vi "DO Control.vi"(9 "DI List_280":string[](array[string]), 10 "s":bool, 11 "Control":string[](array[string])) -> (0 "Feedback":i32[](array[numeric]), 1 "Parameter (Out)":u8 caption="Poll Type", 2 "Control Channel":i32[](array[numeric]), 3 "Poll Time (Out)":u32 caption="Poll Time (ms)" max=600000 step=100, 4 "Tab Control 2":enum32{"Output", "Input"}(ring), 5 "Cancel":bool)   [LabVIEW 2015]
uses:
  Control Button/Exit.ctl
  Control Button/next.ctl
  Galobal variable_TI.vi
panel:
  out "Row":i32
  in  "s 2":bool
  out "Pokayoka Result":cluster{"Sensor Name":string, "Boolean":bool}[](array[cluster]) caption="Pokayoka Status"
  in  "Tab Control":enum32{"Output", "Input"}(tab)
  in  "Control Channel":i32[](listbox)=[7]
  in  "Control":bool
  in  "Feed Back Channel":i32[](listbox)=[0]
  in  "ok":T1
  in  "stop":T2
  # "Control Channel"
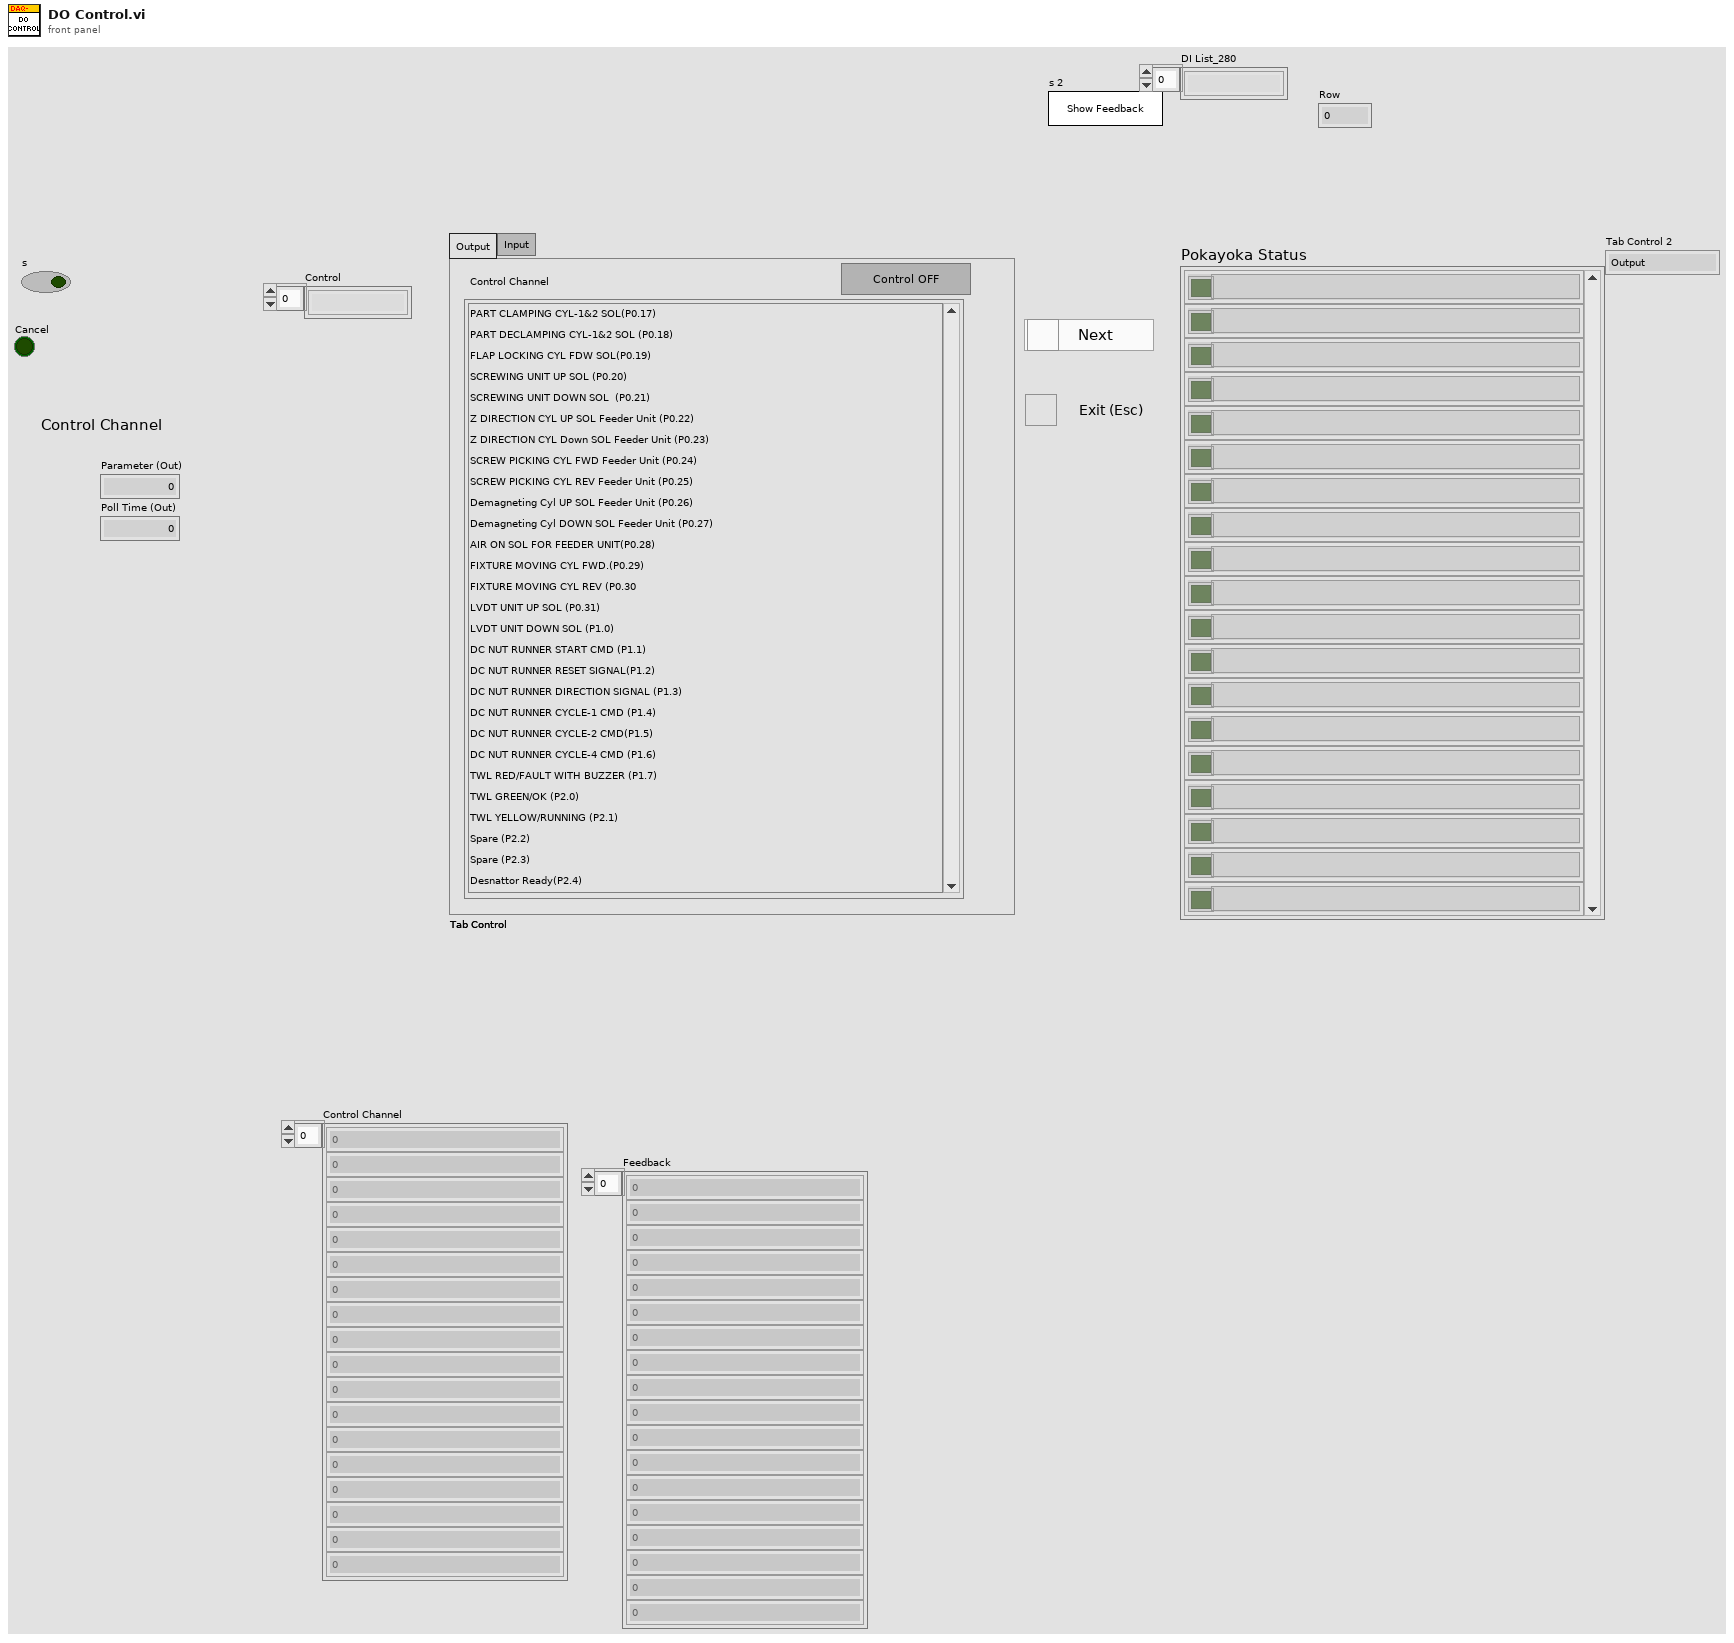
[diagram p1: front panel]
types:
  T1 = typedef "next.ctl" = bool
  T2 = typedef "Exit.ctl" = bool
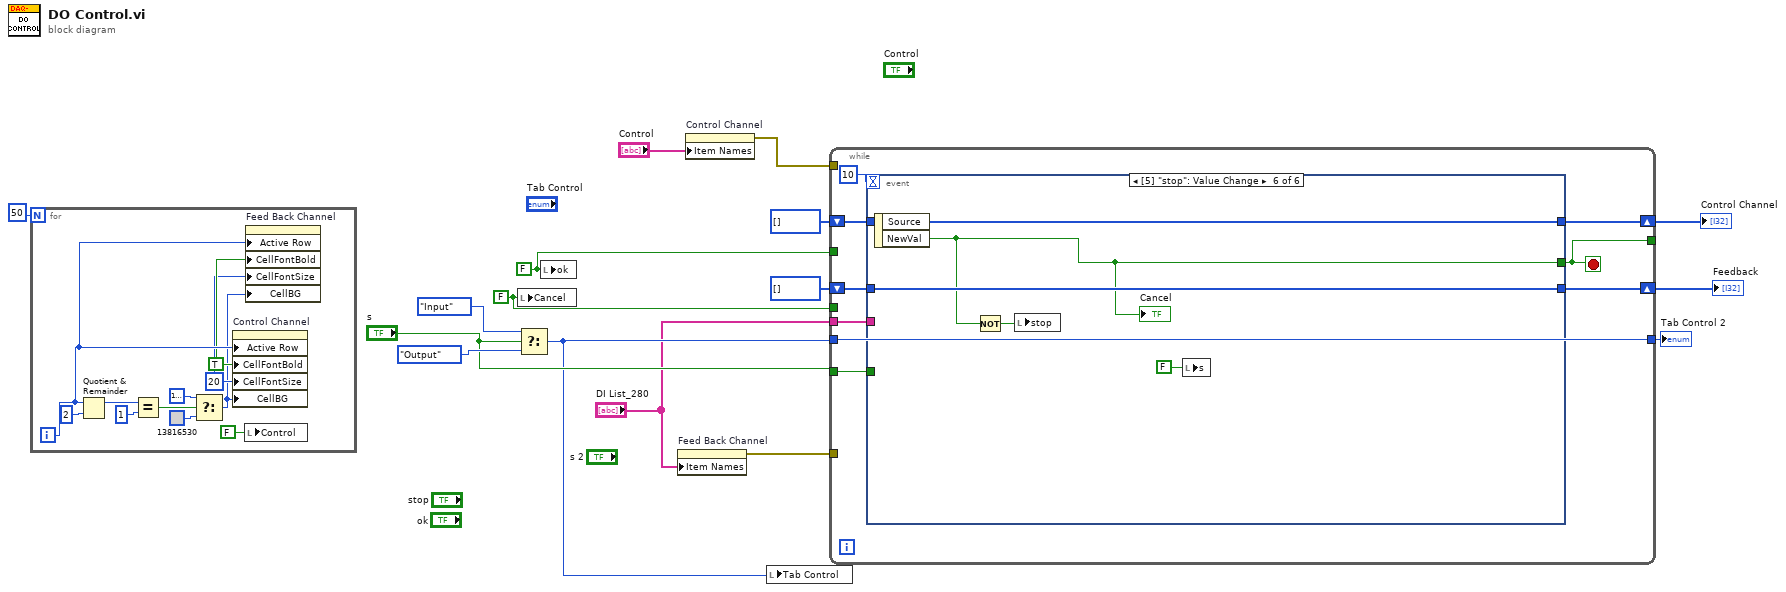
[diagram p0: block diagram]
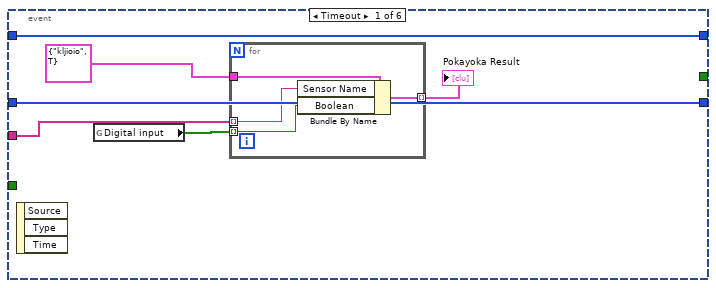
[diagram p2: hidden frame]
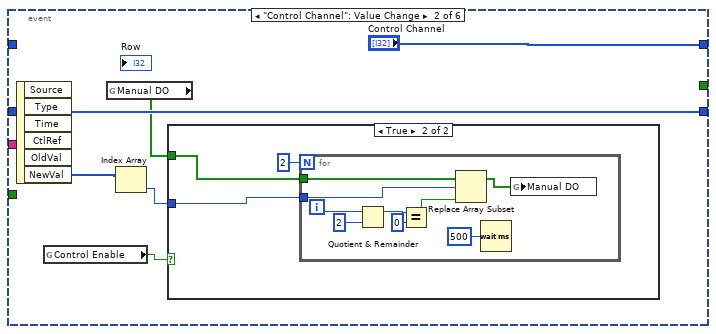
[diagram p3: hidden frame]
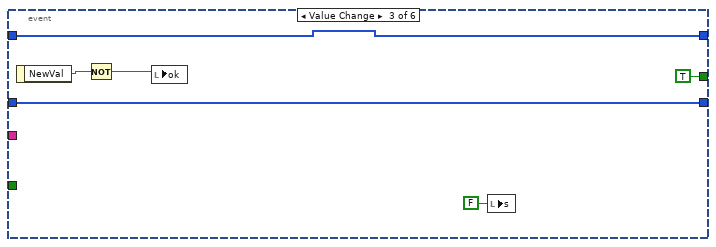
[diagram p5: hidden frame]
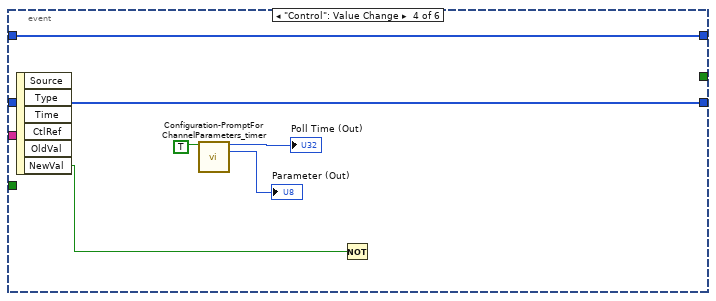
[diagram p6: hidden frame]
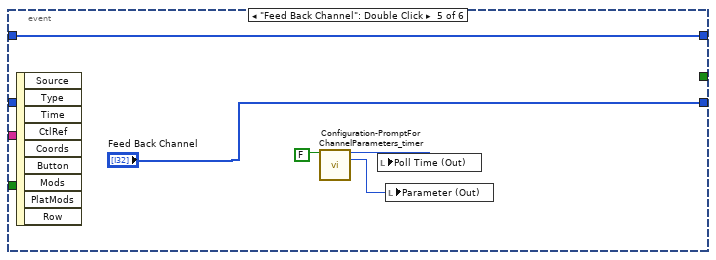
[diagram p7: hidden frame]
diagram:
  w9 = FALSE ("Cancel")
  w10 = FALSE ("ok")
  n1 = for {
    N: 50 -> [_]
    i -> [w21]
    w19 = u32 20 ("Active Row:Cell Font:Size")
    w20 = TRUE ("Active Row:Cell Font:Bold")
    n2 = Quotient & Remainder(x=w21, y=2) -> (x-y*floor(x/y)=w26:i32)  [unwired: 1 out]
    n3 = Equal?(x=w26, y=1) -> (x = y?=w24:bool)
    n4 = Select(t=u32 16777225 ("Color Box"), s=w24, f=u32 13816530 ("Color Box")) -> (s? t:f=w18:u32)
    n5 = property on="Control Channel" class="LstBox (strict)"("Active Row"=w21, "CellFontBold"=w20, "CellFontSize"=w19, "CellBG"=w18) -> ()  [unwired: 2 in, 2 out]
    n6 = local write "Control"(FALSE ("Control")) -> ()
    n7 = property on="Feed Back Channel" class="LstBox (strict)"("Active Row"=w21, "CellFontBold"=w20, "CellFontSize"=w19, "CellBG"=w18) -> ()  [unwired: 2 in, 2 out]
  }
  n8 = local write "Cancel"(w9) -> ()
  n9 = Select(t=enum32{"Output", "Input"}."Input" ("Tab Control"), s="s", f=enum32{"Output", "Input"}."Output" ("Tab Control")) -> (s? t:f=w12:enum32{"Output", "Input"})
  n10 = local write "ok"(w10) -> ()
  n11 = property on="Feed Back Channel" class="LstBox (strict)"("Item Names"="DI List_280") -> (error out=w7:errorcluster)  [unwired: 2 in, 1 out]
  n12 = property on="Control Channel" class="LstBox (strict)"("Item Names"="Control") -> (error out=w5:errorcluster)  [unwired: 2 in, 1 out]
  n13 = local write "Tab Control"(w12) -> ()
  n14 = while {
    tunnel: w12 -> [w28]
    tunnel: "s" -> [w35]
    tunnel: w10 -> [_]
    tunnel: [w33] -> _
    tunnel: w9 -> [_]
    shift-right: [w36] -> w16
    shift-left: i32[] [] ("Control Channel") -> [w32]
    shift-right: [w34] -> w11
    shift-left: i32[] [] ("Feed Back Channel") -> [w31]
    tunnel: "DI List_280" -> [w30]
    tunnel: w7 -> [_]
    tunnel: w5 -> [_]
    tunnel: [w28] -> w3
    stop <- w33 stop-if-true
    n15 = event shown="[5] \"stop\": Value Change" {
      selector: _ -> [_ _ _ _ _ _]
      dyn-events: _ -> [_ _ _ _ _ _]
      timeout: 10 -> [_ _ _ _ _ _]
      tunnel: [w42 "Control Channel" w69 w76 w78 w85] -> w36
      tunnel: [_ _ T2 TRUE ("NewVal") _ _ w83] -> w33
      tunnel: w35 -> [_ _ _ _ _ _]
      tunnel: [w41 w51 w68 w75 "Feed Back Channel" w84] -> w34
      tunnel: w32 -> [w42 _ w69 w76 w78 w85]
      tunnel: w31 -> [w41 w51 w68 w75 _ w84]
      tunnel: w30 -> [w38 _ _ _ _ _]
      event Timeout {
        n16 = event-data() -> ()  [unwired: 1 in, 3 out]
        n17 = global read "Galobal variable_TI.vi" "Digital input"() -> (w40:bool[])
        n18 = for {
          tunnel: w38 -> [w45] mode=indexing
          tunnel: cluster{"Sensor Name":string, "Boolean":bool} {"Sensor Name"="kljioio", "Boolean"=TRUE} ("Cluster") -> [w46]
          tunnel: [w44] -> w37 mode=indexing
          tunnel: w40 -> [w43] mode=indexing
          n19 = Bundle By Name(cluster=w46, "Sensor Name"=w45, "Boolean"=w43) -> (w44:cluster{"Sensor Name":string, "Boolean":bool})
        }
        "Pokayoka Result" <- w37
      }
      event "Control Channel": Value Change {
        n20 = event-data() -> ("NewVal"=w50:i32[])  [unwired: 1 in, 5 out]
        n21 = global read "Galobal variable_TI.vi" "Control Enable"() -> (w48:bool)
        n22 = global read "Galobal variable_TI.vi" "Manual DO"() -> (w47:bool[])
        n23 = Index Array(array=w50) -> (element=w49:i32)  [unwired: 1 in]
        n24 = case shown="True" w48 {
          tunnel: w49 -> [_ w53]
          tunnel: w47 -> [_ w54]
          frame False {
          }
          frame True {
            n25 = for {
              N: 2 -> [_]
              tunnel: w54 -> [w59]
              tunnel: w53 -> [w57]
              i -> [w64]
              n26 = Quotient & Remainder(x=w64, y=2) -> (x-y*floor(x/y)=w62:i32)  [unwired: 1 out]
              n27 = Equal?(x=w62, y=0) -> (x = y?=w58:bool)
              n28 = Replace Array Subset(array=w59, new element=w58, index=w57) -> (w56:bool[])
              n29 = Wait (ms)(milliseconds to wait=u32 500) -> ()  [unwired: 1 out]
              n30 = global write "Galobal variable_TI.vi" "Manual DO"(w56) -> ()
            }
          }
        }
      }
      event Value Change {
        n31 = event-data() -> ("NewVal"=w66:T1)  [unwired: 1 in]
        n32 = Not(x=w66) -> (.not. x?=w65:T1)
        n33 = local write "ok"(w65) -> ()
        n34 = local write "s"(FALSE ("s")) -> ()
      }
      event "Control": Value Change {
        n35 = event-data() -> ("NewVal"=w71:bool)  [unwired: 1 in, 5 out]
        n36 = call "Configuration-PromptForChannelParameters_timer.vi"("Control/Feedback\n(Default: False = Feedback)"=TRUE ("Control/Feedback\n(Default: False = Feedback)")) -> ("Poll Time (Out)"=→"Poll Time (Out)":u32, "Parameter (Out)"=→"Parameter (Out)":u8)  [unwired: 13 in]
        n37 = Not(x=w71) -> ()  [unwired: 1 out]
      }
      event "Feed Back Channel": Double Click {
        n38 = event-data() -> ()  [unwired: 1 in, 9 out]
        n39 = call "Configuration-PromptForChannelParameters_timer.vi"("Control/Feedback\n(Default: False = Feedback)"=FALSE ("Control/Feedback\n(Default: False = Feedback)")) -> ("Poll Time (Out)"=w80:u32, "Parameter (Out)"=w79:u8)  [unwired: 13 in]
        n40 = local write "Poll Time (Out)"(w80) -> ()
        n41 = local write "Parameter (Out)"(w79) -> ()
      }
      event Value Change {
        n42 = event-data() -> ("NewVal"=w83:T2)  [unwired: 1 in, 1 out]
        "Cancel" <- w83
        n43 = Not(x=w83) -> (.not. x?=w82:T2)
        n44 = local write "stop"(w82) -> ()
        n45 = local write "s"(FALSE ("s")) -> ()
      }
    }
  }
  "Control Channel" <- w16
  "Feedback" <- w11
  "Tab Control 2" <- w3
